vi "Initialize.vi"(8 "error in":errorcluster, 9 "result":bool, 10 "time/date":timestamp=timestamp(3230114789.968 s since 1904-01-01)) -> (0 "error out":errorcluster, 3 "test results out":refnum<class "Test Results.lvclass">)   [LabVIEW 2020, in "Test Results.lvclass"]
doc: "This VI initializes the data members of the class \"Test Results.\""
uses:
  Test Results.lvclass
  Test Results.lvclass/Test Results.ctl
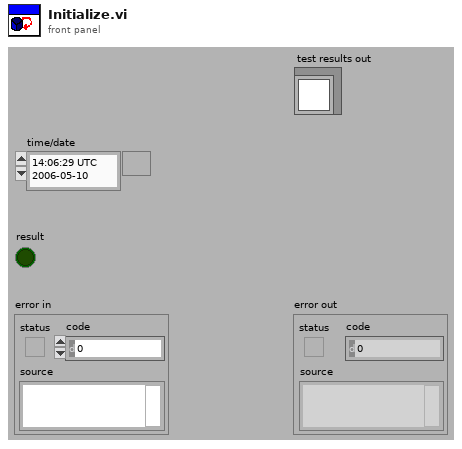
[diagram p1: front panel]
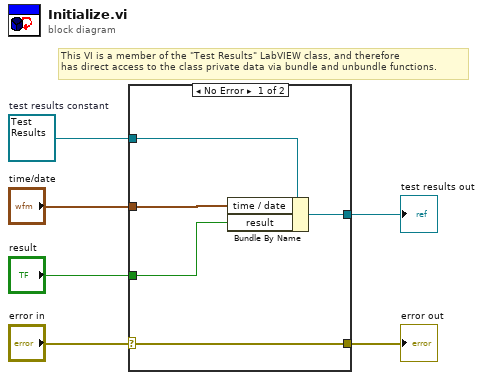
[diagram p0: block diagram]
diagram:
  w6 = refnum<class "Test Results.lvclass"> refnum  # test results constant
  # "This VI is a member of the \"Test Results\" LabVIEW class, and therefore\nhas direct access to the class private data via bundle and unbundle functions."
  n1 = case shown="No Error" "error in" {
    selector: "error in" -> [w7 w13]
    tunnel: w6 -> [w11 w12]
    tunnel: [w10 w12] -> w5
    tunnel: "time/date" -> [w9 _]
    tunnel: "result" -> [w8 _]
    tunnel: [w7 w13] -> w1
    frame No Error {
      n2 = Bundle By Name(cluster=w11, "time / date"=w9, "result"=w8) -> (w10:refnum<class "Test Results.lvclass">)
    }
    frame Error {
    }
  }
  "test results out" <- w5
  "error out" <- w1
